vi "obstructed in left.vi"(8 "error in (no error)":errorcluster, 11 "KNR in":T2) -> (0 "error out":errorcluster, 3 "KNR out":T2, 4 "DC Position Offset":i32)   [LabVIEW 2013]
uses:
  <userlib>/KNR OS 3.0 LabVIEW Toolkit/Type Definition/KNR3 Reference.ctl
  <userlib>/_FPGA Interface Advanced Tools/FPGA Interface Base/FPGA Interface Base.lvclass
  <userlib>/KNR OS 3.0 LabVIEW Toolkit/Type Definition/Resource.ctl
  Global 1.vi
panel:
  out "处理前":T1(plugin-control)
  out "最右边的坐标":dbl[][](array[numeric])
  out "处理后":T1(plugin-control)
  out "Error(deg)":ext
  in  "STOP":bool
  out "CM":dbl
  out "e pix":dbl
  out "Aim":dbl
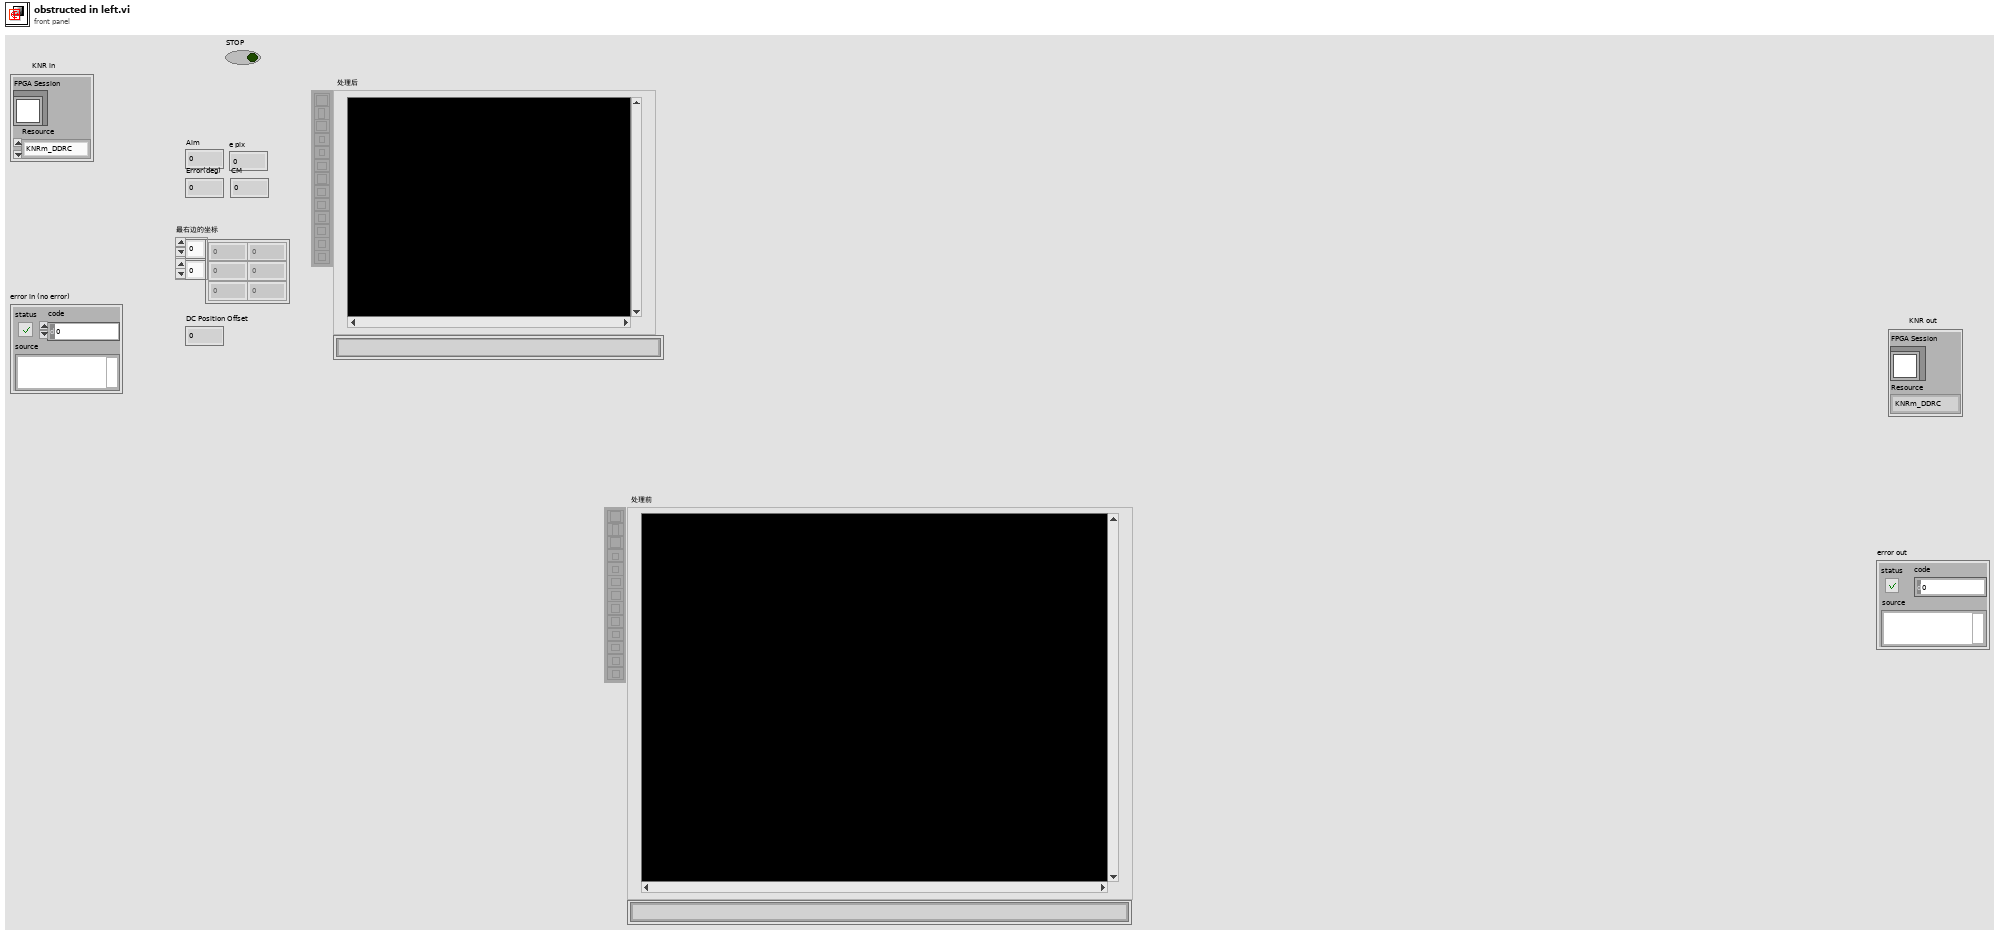
[diagram p1: front panel]
types:
  T1 = typedef "IMAQ Image.ctl" = refnum<image>
  T2 = typedef "KNR3 Reference.ctl" = cluster{"FPGA Session":refnum<class "FPGA Interface Base.lvclass">, "Resource":T3}
  T3 = typedef "Resource.ctl" = enum16{"KNRm_DDRC", "KNRm_DDDD", "KNRm_DDDR", "KNRm_DDDC", "KNR"}
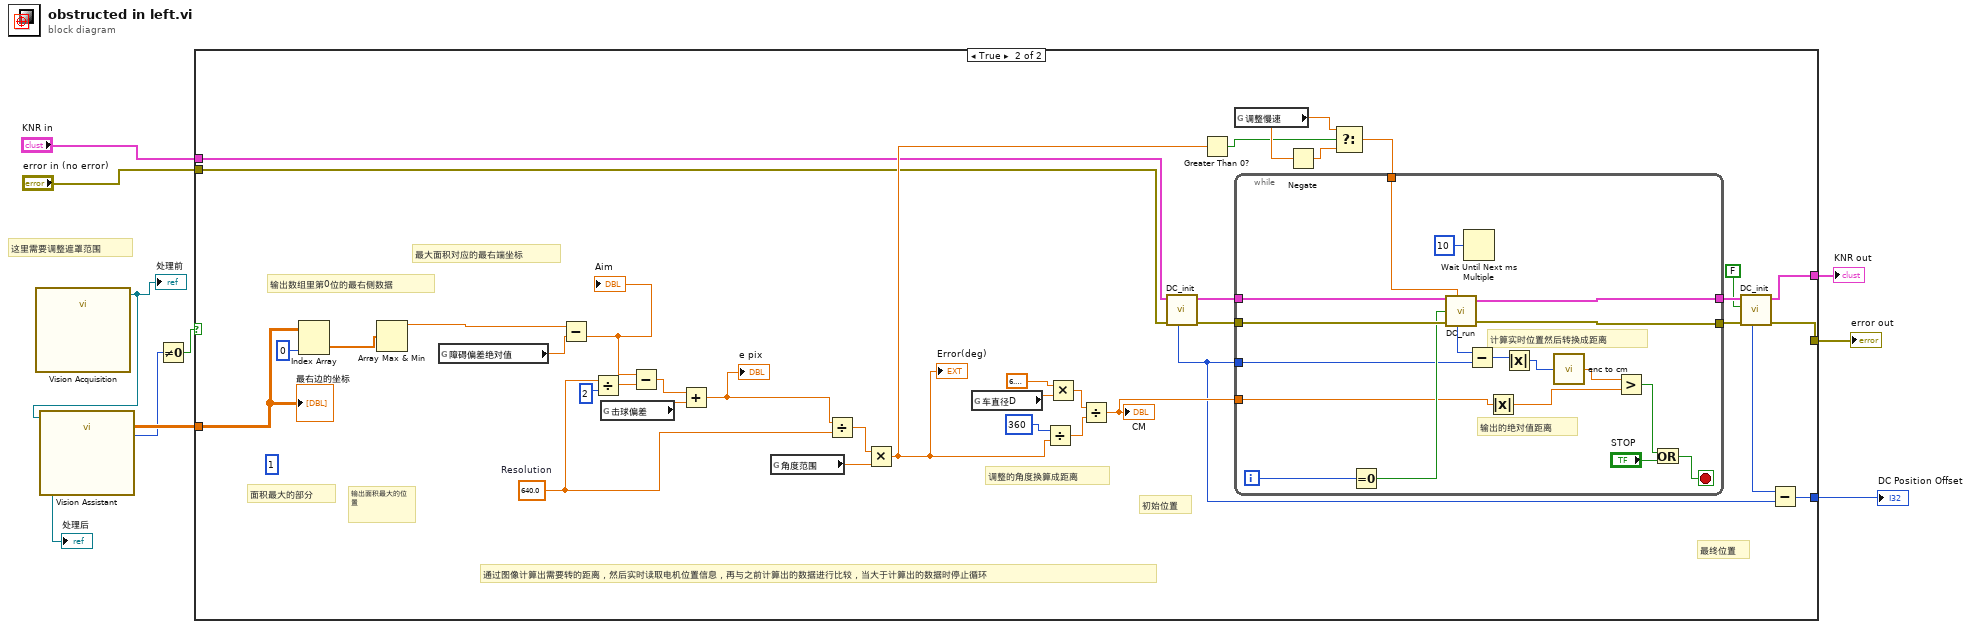
[diagram p0: block diagram]
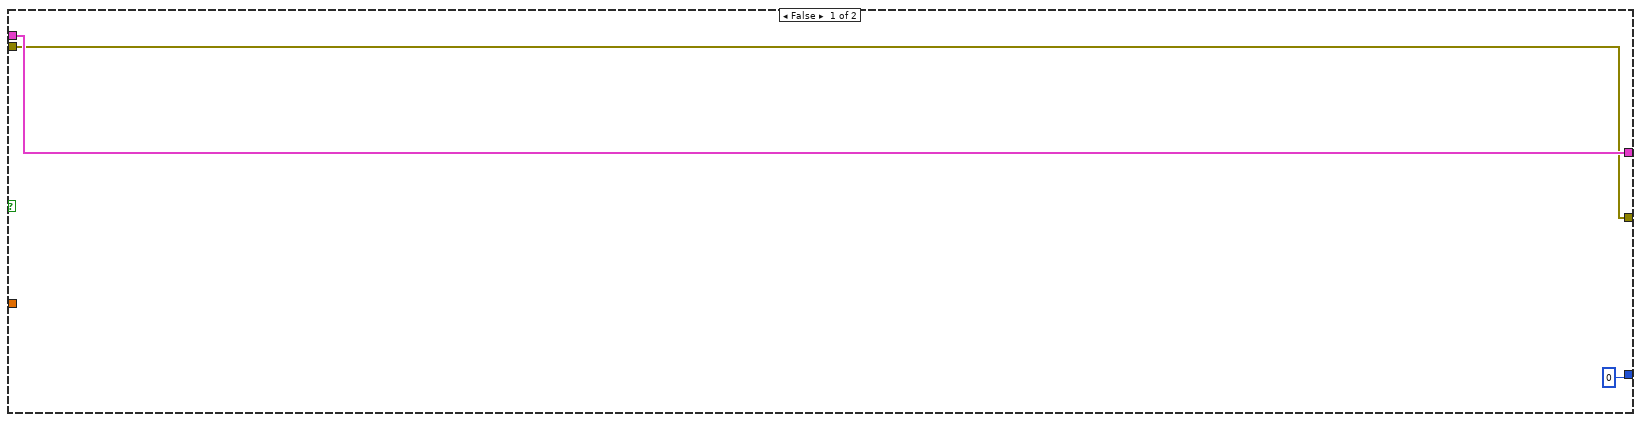
[diagram p2: hidden frame]
diagram:
  # "这里需要调整遮罩范围"
  n1 = call "Vision Acquisition"() -> ("Image Out"=w1:T1)  [unwired: 26 in, 1 out]
  "处理前" <- w1
  n2 = call "Vision Assistant"("Image In"=w1) -> ("Image Out"=→"处理后":T1, "Particle Measurements (Pixels) (Particle Analysis 1)"=w7:dbl[][], "Number of Particles (Particle Analysis 1)"=w4:i32)  [unwired: 23 in, 1 out]
  n3 = Not Equal To 0?(x=w4) -> (x != 0?=w5:bool)
  n4 = case shown="True" w5 {
    tunnel: [w13 w24] -> w10
    tunnel: [w12 w23] -> w9
    tunnel: w7 -> [_ w21]
    tunnel: [0 w20] -> w6
    tunnel: "KNR in" -> [w13 w19]
    tunnel: "error in (no error)" -> [w12 w18]
    frame False {
    }
    frame True {
      (unwired) 1 ("disabled index (col)")
      w34 = 640.0  # Resolution
      # "最终位置"
      # "最大面积对应的最右端坐标"
      # "面积最大的部分"
      # "输出面积最大的位置"
      # "输出数组里第0位的最右侧数据"
      # "调整的角度换算成距离"
      # "初始位置"
      # "通过图像计算出需要转的距离，然后实时读取电机位置信息，再与之前计算出的数据进行比较，当大于计算出的数据时停止循环"
      n5 = Index Array(array=w21, index (col)=0 ("disabled index (col)")) -> (element=w16:dbl[])  [unwired: 1 in]
      n6 = Array Max & Min(array=w16) -> (max value=w15:dbl)  [unwired: 3 out]
      n7 = global read "Global 1.vi" "障碍偏差绝对值"() -> (w14:dbl)
      n8 = Subtract(x=w15, y=w14) -> (x-y=w17:dbl)
      "Aim" <- w17
      n9 = Divide(x=w34, y=2) -> (x/y=w33:dbl)
      n10 = global read "Global 1.vi" "击球偏差"() -> (w49:dbl)
      n11 = Subtract(x=w17, y=w33) -> (x-y=w50:dbl)
      n12 = Add(x=w50, y=w49) -> (x+y=w46:dbl)
      "e pix" <- w46
      n13 = global read "Global 1.vi" "角度范围"() -> (w48:dbl)
      n14 = Divide(x=w46, y=w34) -> (x/y=w47:dbl)
      n15 = Multiply(x=w47, y=w48) -> (x*y=w27:dbl)
      "Error(deg)" <- w27
      n16 = global read "Global 1.vi" "车直径D"() -> (w43:dbl)
      n17 = Divide(x=360, y=w27) -> (x/y=w41:dbl)
      n18 = Multiply(x=6.283185307179586, y=w43) -> (x*y=w42:dbl)
      n19 = Divide(x=w42, y=w41) -> (x/y=w38:dbl)
      "CM" <- w38
      n20 = call "DC_init.vi"("error in (no error)"=w18, "KNR in"=w19) -> ("error out"=w39:errorcluster, "KNR out"=w40:T2, "output\nPosition_1"=w31:i32)  [unwired: 6 in, 1 out]
      n21 = Greater Than 0?(x=w27) -> (x > 0?=w28:bool)
      n22 = global read "Global 1.vi" "调整慢速"() -> (w29:dbl)
      n23 = Negate(x=w29) -> (-x=w30:dbl)
      n24 = Select(t=w29, s=w28, f=w30) -> (s? t:f=w26:dbl)
      n25 = while {
        tunnel: w40 -> [w68]
        tunnel: w39 -> [w67]
        tunnel: [w66] -> w37
        tunnel: [w65] -> w36
        tunnel: w38 -> [w56]
        tunnel: w31 -> [w53]
        tunnel: w26 -> [w51]
        i -> [w59]
        stop <- w62 stop-if-true
        # "输出的绝对值距离"
        # "计算实时位置然后转换成距离"
        n26 = Equal To 0?(x=w59) -> (x = 0?=w58:bool)
        n27 = call "DC_run.vi"("KNR in"=w68, "speed_1"=w51, "reinitialize? (F)"=w58, "error in (no error)"=w67) -> ("Position_1"=w52:i32, "KNR out"=w66:T2, "error out"=w65:errorcluster)  [unwired: 2 in, 1 out]
        n28 = Wait Until Next ms Multiple(millisecond multiple=u32 10) -> ()  [unwired: 1 out]
        n29 = Subtract(x=w52, y=w53) -> (x-y=w64:i32)
        n30 = Absolute Value(x=w56) -> (abs(x)=w63:dbl)
        n31 = Absolute Value(x=w64) -> (abs(x)=w55:i32)
        n32 = call "enc to cm.vi"("E"=w55) -> ("CM"=w54:dbl)  [unwired: 1 in]
        n33 = Greater?(x=w54, y=w63) -> (0:w61:bool)
        n34 = Or(x=w61, y="STOP") -> (x .or. y?=w62:bool)
      }
      n35 = call "DC_init.vi"("error in (no error)"=w36, "Enable Motor(T)"=FALSE, "KNR in"=w37) -> ("error out"=w23:errorcluster, "KNR out"=w24:T2, "output\nPosition_1"=w25:i32)  [unwired: 5 in, 1 out]
      n36 = Subtract(x=w25, y=w31) -> (x-y=w20:i32)
      "最右边的坐标" <- w21
    }
  }
  "error out" <- w9
  "KNR out" <- w10
  "DC Position Offset" <- w6
